vi "VectorNav parse QMA.vi"(11 "input data":u8) -> ()   [LabVIEW 2010]
uses:
  VectorNav parse QMA state typedef.vi
  vectornav data.vi
panel:
  out "number":dbl
  out "data array length":u8
  out "data array":u8[](array[numeric])
  # "change i can believe in!"
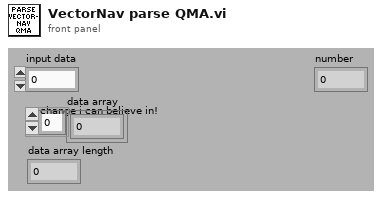
[diagram p1: front panel]
types:
  T1 = typedef "VectorNav parse QMA state typedef.vi" = enum16{"wait for $", "confirm command", "q[0] of quaternion", "q[1] of quaternion", "q[2] of quaternion", "q[3] of quaternion (scalar term)", "X-Axis Magnetic", "Y-Axis Magnetic", "Z-Axis Magnetic", "X-Axis Acceleration", "Y-Axis-Acceleration", "Z-Axis-Acceleration", "Checksum"}
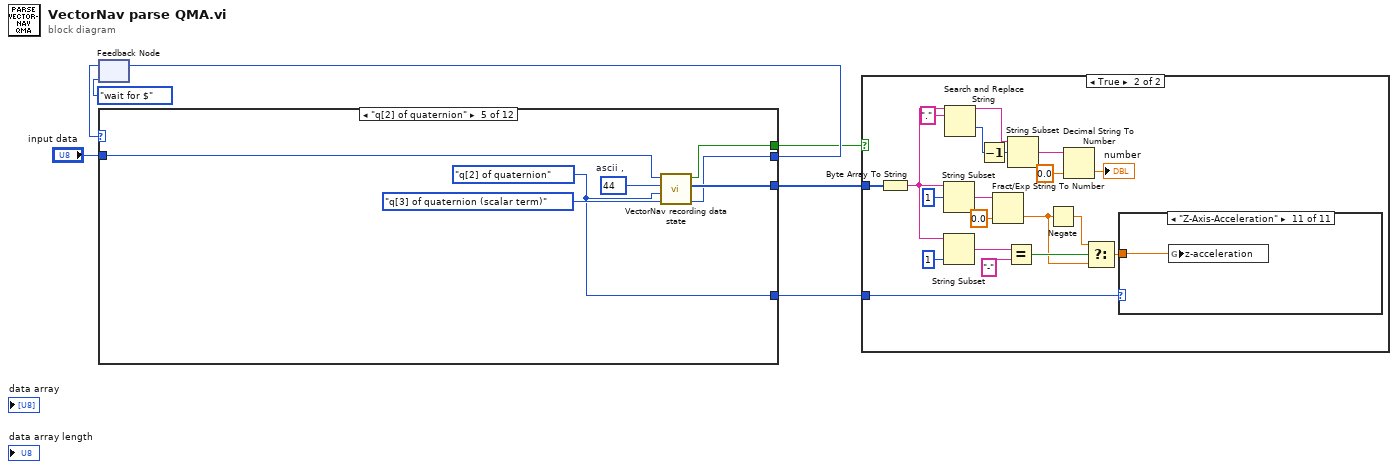
[diagram p0: block diagram]
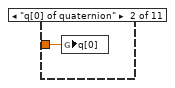
[diagram p4: hidden frame]
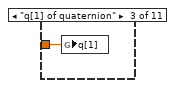
[diagram p5: hidden frame]
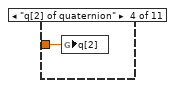
[diagram p6: hidden frame]
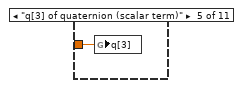
[diagram p7: hidden frame]
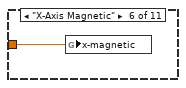
[diagram p8: hidden frame]
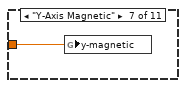
[diagram p9: hidden frame]
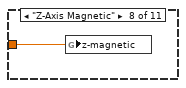
[diagram p10: hidden frame]
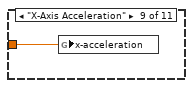
[diagram p11: hidden frame]
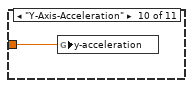
[diagram p12: hidden frame]
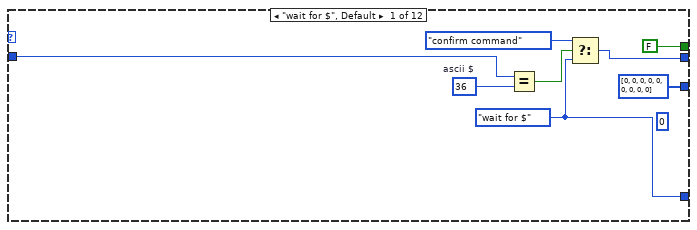
[diagram p13: hidden frame]
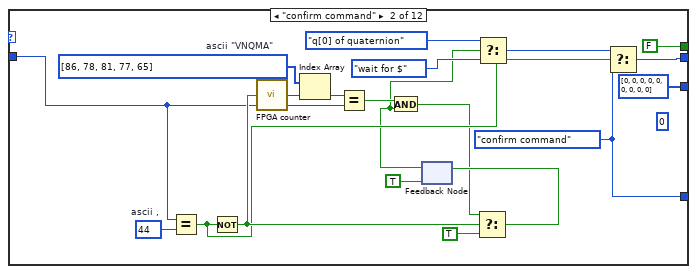
[diagram p14: hidden frame]
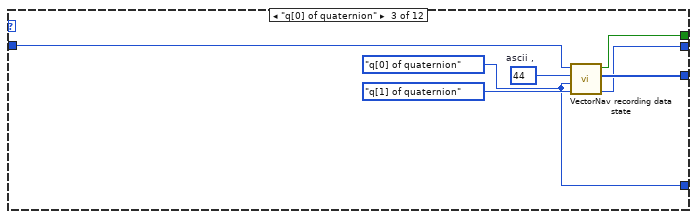
[diagram p15: hidden frame]
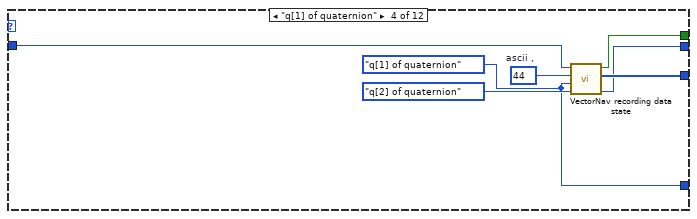
[diagram p16: hidden frame]
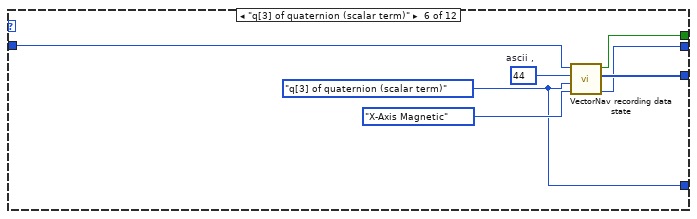
[diagram p17: hidden frame]
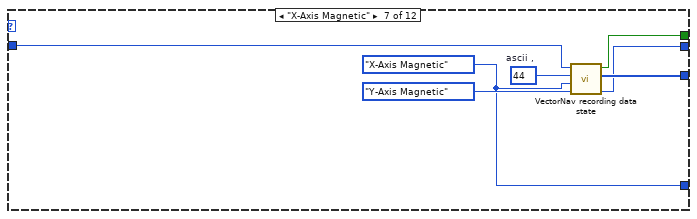
[diagram p18: hidden frame]
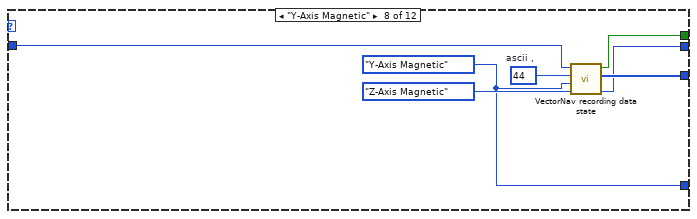
[diagram p19: hidden frame]
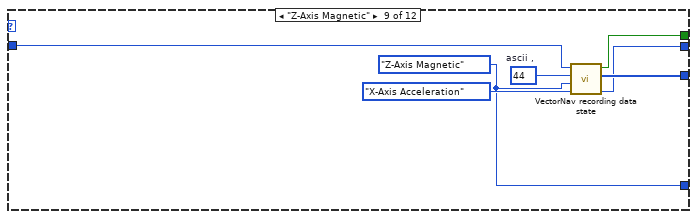
[diagram p20: hidden frame]
diagram:
  n1 = feedback #1(VectorNav_parse_QMA_state_typedef.vi."wait for $" ("Enum")) -> (w6:T1)
  n2 = case shown="\"q[2] of quaternion\"" w6 {
    tunnel: "input data" -> [w15 w24 w42 w49 w56 w63 w70 w77 w84 w91 w98 w105]
    tunnel: [w11 w31 w39 w45 w52 w58 w65 w72 w79 w86 w93 w101] -> w4
    tunnel: [u8[] [0, 0, 0, 0, 0, 0, 0, 0, 0] ("Array") u8[] [0, 0, 0, 0, 0, 0, 0, 0, 0] ("Array") w40 w46 w53 w59 w66 w73 w80 w87 w94 w102] -> w2
    tunnel: [FALSE FALSE w41 w47 w54 w60 w67 w74 w81 w88 w95 w103] -> w3
    tunnel: [w8 w16 w36 w43 w50 w57 w64 w71 w78 w85 w92 w99] -> w1
    frame "wait for $", Default {
      (unwired) u8 0 ("count")
      w8 = VectorNav_parse_QMA_state_typedef.vi."wait for $" ("Enum")
      w14 = u8 36  # ascii $
      n3 = Equal?(x=w15, y=w14) -> (x = y?=w13:bool)
      n4 = Select(t=VectorNav_parse_QMA_state_typedef.vi."confirm command" ("Enum"), s=w13, f=w8) -> (s? t:f=w11:T1)
    }
    frame "confirm command" {
      (unwired) u8 0 ("count")
      w22 = u8[] [86, 78, 81, 77, 65]  # ascii "VNQMA"
      w16 = VectorNav_parse_QMA_state_typedef.vi."confirm command" ("Enum")
      w35 = u8 44  # ascii ,
      n5 = Equal?(x=w24, y=w35) -> (x = y?=w23:bool)
      n6 = Not(x=w23) -> (.not. x?=w28:bool)
      n7 = call "FPGA counter.vi"("no reset?"=w28) -> ("count"=w25:u8)
      n8 = Index Array(array=w22, index=w25) -> (element=w26:u8)
      n9 = Equal?(x=w26, y=w24) -> (x = y?=w27:bool)
      n10 = feedback #2(TRUE ("f")) -> (w17:bool)
      n11 = And(x=w27, y=w17) -> (x .and. y?=w20:bool)
      n12 = Select(t=w20, s=w28, f=TRUE) -> (s? t:f=w21:bool)
      n13 = feedback-in #2(w21) -> ()
      n14 = Select(t=VectorNav_parse_QMA_state_typedef.vi."q[0] of quaternion" ("Enum"), s=w17, f=VectorNav_parse_QMA_state_typedef.vi."wait for $" ("Enum")) -> (s? t:f=w32:T1)
      n15 = Select(t=w32, s=w23, f=w16) -> (s? t:f=w31:T1)
    }
    frame "q[0] of quaternion" {
      w38 = u8 44  # ascii ,
      w36 = VectorNav_parse_QMA_state_typedef.vi."q[0] of quaternion" ("current state")
      n16 = call "VectorNav recording data state.vi"("next state"=VectorNav_parse_QMA_state_typedef.vi."q[1] of quaternion", "current state"=w36, "stop character"=w38, "input data"=w42) -> ("state to transition to"=w39:T1, "recorded data array"=w40:u8[], "Boolean"=w41:bool)  [unwired: 1 out]
    }
    frame "q[1] of quaternion" {
      w48 = u8 44  # ascii ,
      w43 = VectorNav_parse_QMA_state_typedef.vi."q[1] of quaternion" ("current state")
      n17 = call "VectorNav recording data state.vi"("next state"=VectorNav_parse_QMA_state_typedef.vi."q[2] of quaternion", "current state"=w43, "stop character"=w48, "input data"=w49) -> ("state to transition to"=w45:T1, "recorded data array"=w46:u8[], "Boolean"=w47:bool)  [unwired: 1 out]
    }
    frame "q[2] of quaternion" {
      w55 = u8 44  # ascii ,
      w50 = VectorNav_parse_QMA_state_typedef.vi."q[2] of quaternion" ("current state")
      n18 = call "VectorNav recording data state.vi"("next state"=VectorNav_parse_QMA_state_typedef.vi."q[3] of quaternion (scalar term)", "current state"=w50, "stop character"=w55, "input data"=w56) -> ("state to transition to"=w52:T1, "recorded data array"=w53:u8[], "Boolean"=w54:bool)  [unwired: 1 out]
    }
    frame "q[3] of quaternion (scalar term)" {
      w57 = VectorNav_parse_QMA_state_typedef.vi."q[3] of quaternion (scalar term)" ("current state")
      w62 = u8 44  # ascii ,
      n19 = call "VectorNav recording data state.vi"("next state"=VectorNav_parse_QMA_state_typedef.vi."X-Axis Magnetic", "current state"=w57, "stop character"=w62, "input data"=w63) -> ("state to transition to"=w58:T1, "recorded data array"=w59:u8[], "Boolean"=w60:bool)  [unwired: 1 out]
    }
    frame "X-Axis Magnetic" {
      w64 = VectorNav_parse_QMA_state_typedef.vi."X-Axis Magnetic" ("current state")
      w69 = u8 44  # ascii ,
      n20 = call "VectorNav recording data state.vi"("next state"=VectorNav_parse_QMA_state_typedef.vi."Y-Axis Magnetic", "current state"=w64, "stop character"=w69, "input data"=w70) -> ("state to transition to"=w65:T1, "recorded data array"=w66:u8[], "Boolean"=w67:bool)  [unwired: 1 out]
    }
    frame "Y-Axis Magnetic" {
      w71 = VectorNav_parse_QMA_state_typedef.vi."Y-Axis Magnetic" ("current state")
      w75 = u8 44  # ascii ,
      n21 = call "VectorNav recording data state.vi"("next state"=VectorNav_parse_QMA_state_typedef.vi."Z-Axis Magnetic", "current state"=w71, "stop character"=w75, "input data"=w77) -> ("state to transition to"=w72:T1, "recorded data array"=w73:u8[], "Boolean"=w74:bool)  [unwired: 1 out]
    }
    frame "Z-Axis Magnetic" {
      w78 = VectorNav_parse_QMA_state_typedef.vi."Z-Axis Magnetic" ("current state")
      w83 = u8 44  # ascii ,
      n22 = call "VectorNav recording data state.vi"("next state"=VectorNav_parse_QMA_state_typedef.vi."X-Axis Acceleration", "current state"=w78, "stop character"=w83, "input data"=w84) -> ("state to transition to"=w79:T1, "recorded data array"=w80:u8[], "Boolean"=w81:bool)  [unwired: 1 out]
    }
    frame "X-Axis Acceleration" {
      w85 = VectorNav_parse_QMA_state_typedef.vi."X-Axis Acceleration" ("current state")
      w90 = u8 44  # ascii ,
      n23 = call "VectorNav recording data state.vi"("next state"=VectorNav_parse_QMA_state_typedef.vi."Y-Axis-Acceleration", "current state"=w85, "stop character"=w90, "input data"=w91) -> ("state to transition to"=w86:T1, "recorded data array"=w87:u8[], "Boolean"=w88:bool)  [unwired: 1 out]
    }
    frame "Y-Axis-Acceleration" {
      w92 = VectorNav_parse_QMA_state_typedef.vi."Y-Axis-Acceleration" ("current state")
      w97 = u8 44  # ascii ,
      n24 = call "VectorNav recording data state.vi"("next state"=VectorNav_parse_QMA_state_typedef.vi."Z-Axis-Acceleration", "current state"=w92, "stop character"=w97, "input data"=w98) -> ("state to transition to"=w93:T1, "recorded data array"=w94:u8[], "Boolean"=w95:bool)  [unwired: 1 out]
    }
    frame "Z-Axis-Acceleration" {
      w100 = u8 42  # ascii ,
      w99 = VectorNav_parse_QMA_state_typedef.vi."Z-Axis-Acceleration" ("current state")
      n25 = call "VectorNav recording data state.vi"("next state"=VectorNav_parse_QMA_state_typedef.vi."confirm command", "current state"=w99, "stop character"=w100, "input data"=w105) -> ("state to transition to"=w101:T1, "recorded data array"=w102:u8[], "Boolean"=w103:bool)  [unwired: 1 out]
    }
  }
  n26 = feedback-in #1(w4) -> ()
  n27 = case shown="True" w3 {
    tunnel: w2 -> [_ w125]
    tunnel: w1 -> [_ w106]
    frame False {
    }
    frame True {
      n28 = Byte Array To String(unsigned byte array=w125) -> (string=w114:string)
      n29 = String Subset(string=w114, offset (0)=1 ("length (rest)")) -> (substring=w122:string)  [unwired: 1 in]
      n30 = String Subset(string=w114, length (rest)=1 ("length (rest)")) -> (substring=w120:string)  [unwired: 1 in]
      n31 = Search and Replace String(input string=w114, search string=".") -> (result string=w111:string, offset past replacement=w112:i32)  [unwired: 6 in, 2 out]
      n32 = Decrement(x=w112) -> (x-1=w107:i32)
      n33 = Fract/Exp String To Number(string=w122, default (0 dbl)=0.0 ("default (0 I32)")) -> (number=w116:dbl)  [unwired: 2 in, 1 out]
      n34 = Equal?(x=w120, y="-") -> (x = y?=w118:bool)
      n35 = String Subset(string=w111, offset (0)=w107) -> (substring=w110:string)  [unwired: 1 in]
      n36 = Negate(x=w116) -> (-x=w117:dbl)
      n37 = Decimal String To Number(string=w110, default (0L)=0.0 ("default (0 I32)")) -> (number=→"number":dbl)  [unwired: 1 in, 1 out]
      n38 = Select(t=w117, s=w118, f=w116) -> (s? t:f=w115:dbl)
      n39 = case shown="\"Z-Axis-Acceleration\"" w106 {
        tunnel: w115 -> [_ w126 w127 w128 w129 w130 w131 w132 w133 w134 w135]
        frame "confirm command", Default {
          # "hi"
        }
        frame "q[0] of quaternion" {
          n40 = global write "vectornav data.vi" "q[0]"(w126) -> ()
        }
        frame "q[1] of quaternion" {
          n41 = global write "vectornav data.vi" "q[1]"(w127) -> ()
        }
        frame "q[2] of quaternion" {
          n42 = global write "vectornav data.vi" "q[2]"(w128) -> ()
        }
        frame "q[3] of quaternion (scalar term)" {
          n43 = global write "vectornav data.vi" "q[3]"(w129) -> ()
        }
        frame "X-Axis Magnetic" {
          n44 = global write "vectornav data.vi" "x-magnetic"(w130) -> ()
        }
        frame "Y-Axis Magnetic" {
          n45 = global write "vectornav data.vi" "y-magnetic"(w131) -> ()
        }
        frame "Z-Axis Magnetic" {
          n46 = global write "vectornav data.vi" "z-magnetic"(w132) -> ()
        }
        frame "X-Axis Acceleration" {
          n47 = global write "vectornav data.vi" "x-acceleration"(w133) -> ()
        }
        frame "Y-Axis-Acceleration" {
          n48 = global write "vectornav data.vi" "y-acceleration"(w134) -> ()
        }
        frame "Z-Axis-Acceleration" {
          n49 = global write "vectornav data.vi" "z-acceleration"(w135) -> ()
        }
      }
    }
  }
